vi "Configure sample changer.vi"(7 "ID":i32) -> (3 "ID out":i32)   [LabVIEW 2012]
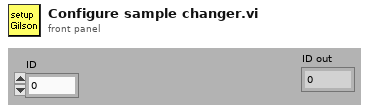
[diagram p1: front panel]
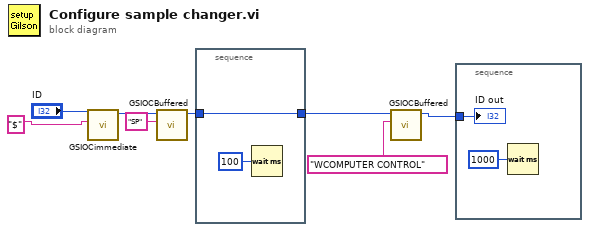
[diagram p0: block diagram]
diagram:
  n1 = call "GSIOCimmediate.vi"("Command"="$", "ID"="ID") -> ("ID out"=w6:i32)  [unwired: 4 in, 1 out]
  n2 = call "GSIOCBuffered.vi"("Command"="SP", "ID"=w6) -> ("ID out"=w1:i32)  [unwired: 4 in, 1 out]
  n3 = stacked-sequence {
    tunnel: [w10] -> w2
    tunnel: w1 -> [w10]
    frame #0 {
      n4 = Wait (ms)(milliseconds to wait=u32 100) -> ()  [unwired: 1 out]
    }
  }
  n5 = call "GSIOCBuffered.vi"("Command"="WCOMPUTER CONTROL", "ID"=w2) -> ("ID out"=w3:i32)  [unwired: 4 in, 1 out]
  n6 = stacked-sequence {
    tunnel: w3 -> [w12]
    frame #0 {
      n7 = Wait (ms)(milliseconds to wait=u32 1000) -> ()  [unwired: 1 out]
      "ID out" <- w12
    }
  }
